vi "Method 3.vi"(10 "My Input":dbl, 11 "Test Actor 1 in":refnum<class "Test Actor 1.lvclass">) -> (2 "My Output":dbl, 3 "Test Actor 1 out":refnum<class "Test Actor 1.lvclass">)   [LabVIEW 2023, in "Test Actor 1.lvlib" / "Test Actor 1.lvclass"]
doc: "My Method Description"
uses:
  Test Actor 1.lvclass
  Test Actor 1.lvclass/Test Actor 1.ctl
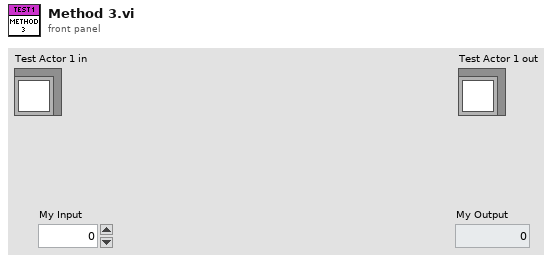
[diagram p1: front panel]
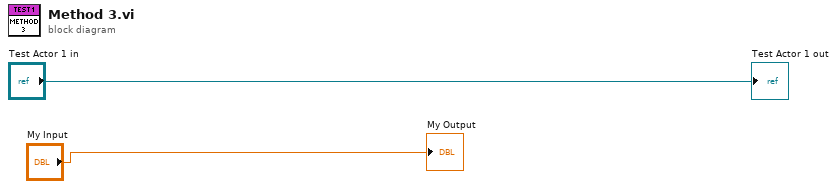
[diagram p0: block diagram]
diagram:
  "Test Actor 1 out" <- "Test Actor 1 in"
  "My Output" <- "My Input"
